vi "LogMessage.vi"(7 "LogLevel":T1=enum."None", 8 "ErrorIn":errorcluster[](array[cluster]), 10 "LogMessage":string) -> (0 "ErrorOut":errorcluster[](array[cluster]))   [LabVIEW 2018]
uses:
  LV_Config/Typedefs/eLogLvl.ctl
  LV_Config/Config.lvclass
  <userlib>/NIST/NISTErrorLib/NISTErrorLib.lvlib
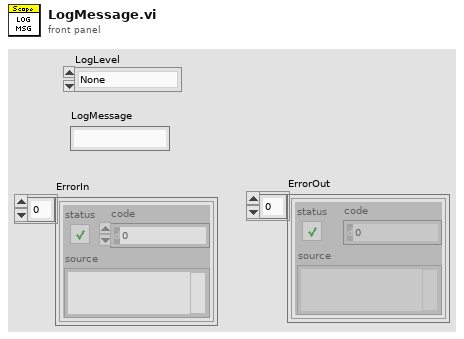
[diagram p1: front panel]
types:
  T1 = typedef "Config_class.lvlib/Config.lvclass/eLogLvl.ctl" = enum16{"Normal", "Verbose", "None"}
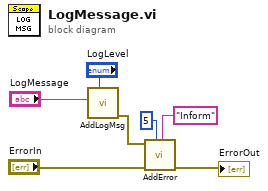
[diagram p0: block diagram]
diagram:
  n1 = call "AddLogMsg.vi"("LogLevel"="LogLevel", "LogMsg"="LogMessage") -> ("error out"=w5:errorcluster)  [unwired: 9 in]
  n2 = call <userlib>:"AddError.vi"("Severity"="Inform", "Priority"=u8 5, "ErrorArray"="ErrorIn", "error in (no error)"=w5) -> ("ErrorArray"=→"ErrorOut":errorcluster[])  [unwired: 6 in, 1 out]
